vi "Signals to JSON 4.vi"() -> ()   [LabVIEW 2021]
uses:
  controls/JSON sigs.ctl
  863f65c0-6e08-4c3b-92ae-c38da8f40fe4.vi
  <vilib>/JDP Science/JSONtext/Variant to JSON Text.vi
  <vilib>/JDP Science/JSONtext/LVClass Serializer/JSONtext LVClass Serializer.lvclass
panel:
  out "JSON string":string
  in  "Signal Sessions":T1
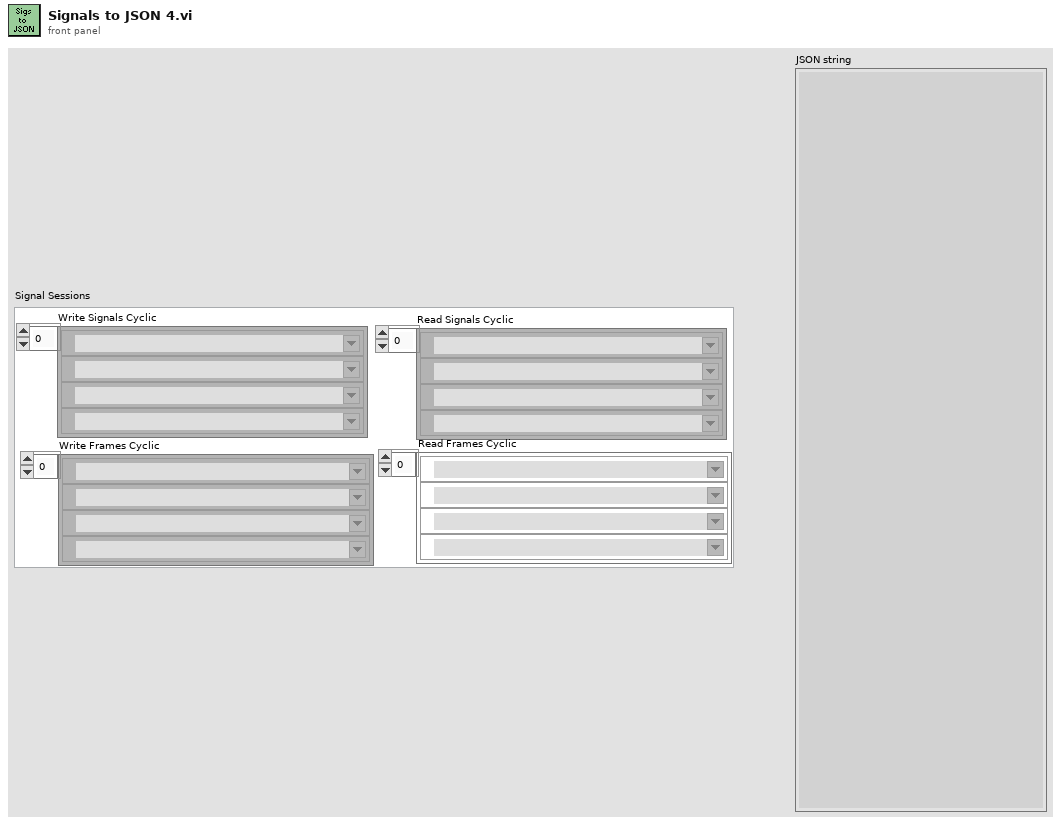
[diagram p1: front panel]
types:
  T1 = typedef "JSON sigs.ctl" = cluster{"Read Signals Cyclic":refnum<k21>[], "Write Signals Cyclic":refnum<k21>[], "Write Frames Cyclic":refnum<k21>[], "Read Frames Cyclic":refnum<k21>[]}
  T2 = cluster{string[], string[], "Write Frames Cyclic":refnum<k21>[]}
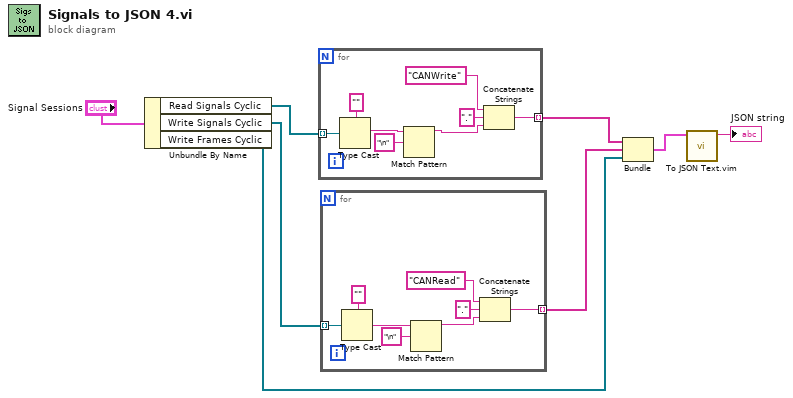
[diagram p0: block diagram]
diagram:
  n1 = Unbundle By Name("Signal Sessions") -> ("Read Signals Cyclic"=w5:refnum<k21>[], "Write Signals Cyclic"=w6:refnum<k21>[], "Write Frames Cyclic"=w1:refnum<k21>[])
  n2 = for {
    tunnel: w5 -> [w10] mode=indexing
    tunnel: [w9] -> w4 mode=indexing
    n3 = Type Cast(type="", x=w10) -> (*(type *) &x=w12:string)
    n4 = Match Pattern(string=w12, regular expression="\n") -> (before substring=w11:string)  [unwired: 1 in, 3 out]
    n5 = Concatenate Strings("CANWrite" ("type"), "." ("string"), w11) -> (w9:string)
  }
  n6 = for {
    tunnel: w6 -> [w23] mode=indexing
    tunnel: [w17] -> w3 mode=indexing
    n7 = Type Cast(type="", x=w23) -> (*(type *) &x=w20:string)
    n8 = Match Pattern(string=w20, regular expression="\n") -> (before substring=w18:string)  [unwired: 1 in, 3 out]
    n9 = Concatenate Strings("CANRead" ("type"), "." ("string"), w18) -> (w17:string)
  }
  n10 = Bundle(w4, w3, "Write Frames Cyclic"=w1) -> (w2:T2)  [unwired: 1 in]
  n11 = call "To JSON Text.vim"("Anything"=w2) -> ("<JSON>"=→"JSON string":string)  [unwired: 9 in, 1 out]
